vi "uTTA_CalcADC_Limits.vi"(8 "Offset Voltage":dbl(slide) min=-2.5 max=2.5 scale=-2.5..2.5 scale format="%#.2pV", 9 "PGA_Setting":u32 max=3, 10 "Channel Number":u32 max=3, 11 "uTTA_CalData":T1(array[cluster])) -> (2 "Range Low End":dbl format="%.3pV", 3 "Range High End":dbl format="%.3pV")   [LabVIEW 2021]
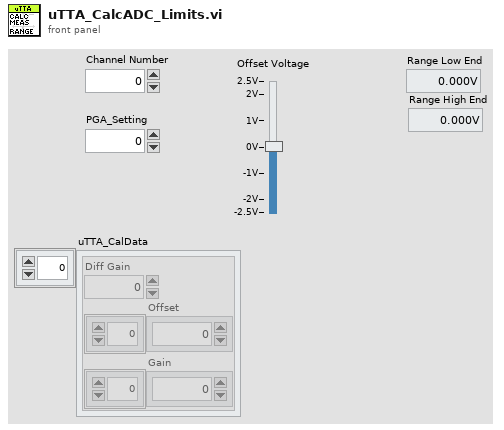
[diagram p1: front panel]
types:
  T1 = cluster{"Diff Gain":dbl, "Offset":dbl[], "Gain":dbl[]}[]
  T2 = cluster{"Diff Gain":dbl, "Offset":dbl[], "Gain":dbl[]}
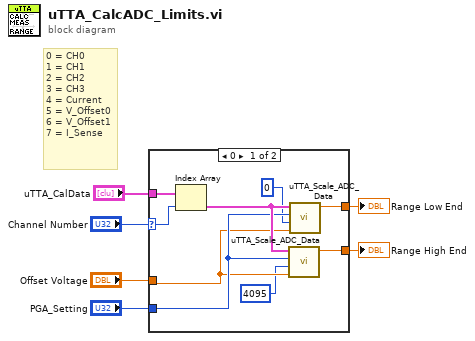
[diagram p0: block diagram]
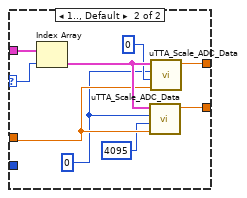
[diagram p2: hidden frame]
diagram:
  # "0 = CH0\n1 = CH1\n2 = CH2\n3 = CH3\n4 = Current\n5 = V_Offset0\n6 = V_Offset1\n7 = I_Sense"
  n1 = case shown="0" "Channel Number" {
    selector: "Channel Number" -> [w14 w23]
    tunnel: "PGA_Setting" -> [w12 _]
    tunnel: "Offset Voltage" -> [w11 w21]
    tunnel: "uTTA_CalData" -> [w15 w24]
    tunnel: [w8 w18] -> w2
    tunnel: [w7 w17] -> w1
    frame 0 {
      n2 = Index Array(array=w15, index=w14) -> (element=w13:T2)
      n3 = call "uTTA_Scale_ADC_Data.vi"("Offset Voltage"=w11, "ADC Value"=4095, "PGA Setting"=w12, "Calibration"=w13) -> ("Scaled Output"=w7:dbl)  [unwired: 3 in]
      n4 = call "uTTA_Scale_ADC_Data.vi"("Offset Voltage"=w11, "ADC Value"=0, "PGA Setting"=w12, "Calibration"=w13) -> ("Scaled Output"=w8:dbl)  [unwired: 3 in]
    }
    frame 1.., Default {
      w16 = 0 ("PGA Setting")
      n5 = Index Array(array=w24, index=w23) -> (element=w22:T2)
      n6 = call "uTTA_Scale_ADC_Data.vi"("Offset Voltage"=w21, "ADC Value"=4095, "PGA Setting"=w16, "Calibration"=w22) -> ("Scaled Output"=w17:dbl)  [unwired: 3 in]
      n7 = call "uTTA_Scale_ADC_Data.vi"("Offset Voltage"=w21, "ADC Value"=0, "PGA Setting"=w16, "Calibration"=w22) -> ("Scaled Output"=w18:dbl)  [unwired: 3 in]
    }
  }
  "Range Low End" <- w2
  "Range High End" <- w1
